vi "Main.vi"() -> ()   [LabVIEW 2019]
uses:
  Motion Profile States.ctl
panel:
  out "CSV (P-V-T)":string[][](table)
  in  "Time between intervals (ms)":dbl=20.0
  in  "Rampdown time (ms)":dbl
  in  "Rampup time (ms)":dbl
  in  "Distance (in)":dbl
  in  "Max Speed (in/sec)":dbl
  out "P-V-A graph":cluster{dbl[], dbl[]}[](graph)
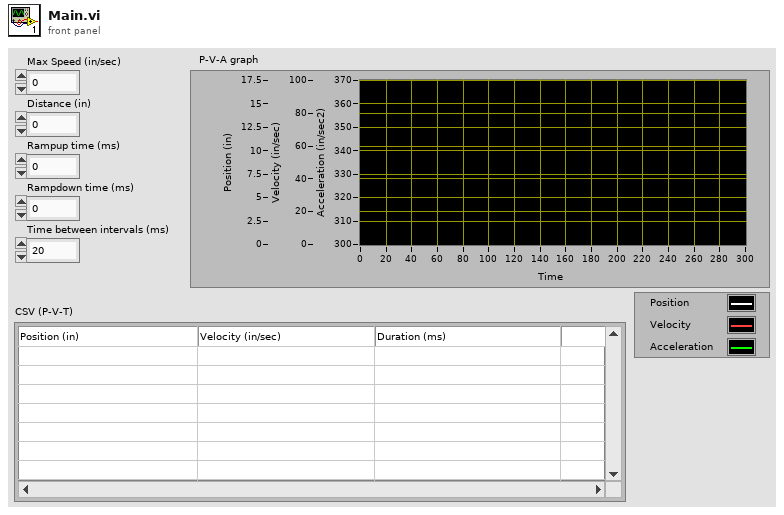
[diagram p1: front panel]
types:
  T1 = typedef "Motion Profile States.ctl" = enum16{"Ramp Up", "ramp down 2", "Steady State", "Ramp Down"}
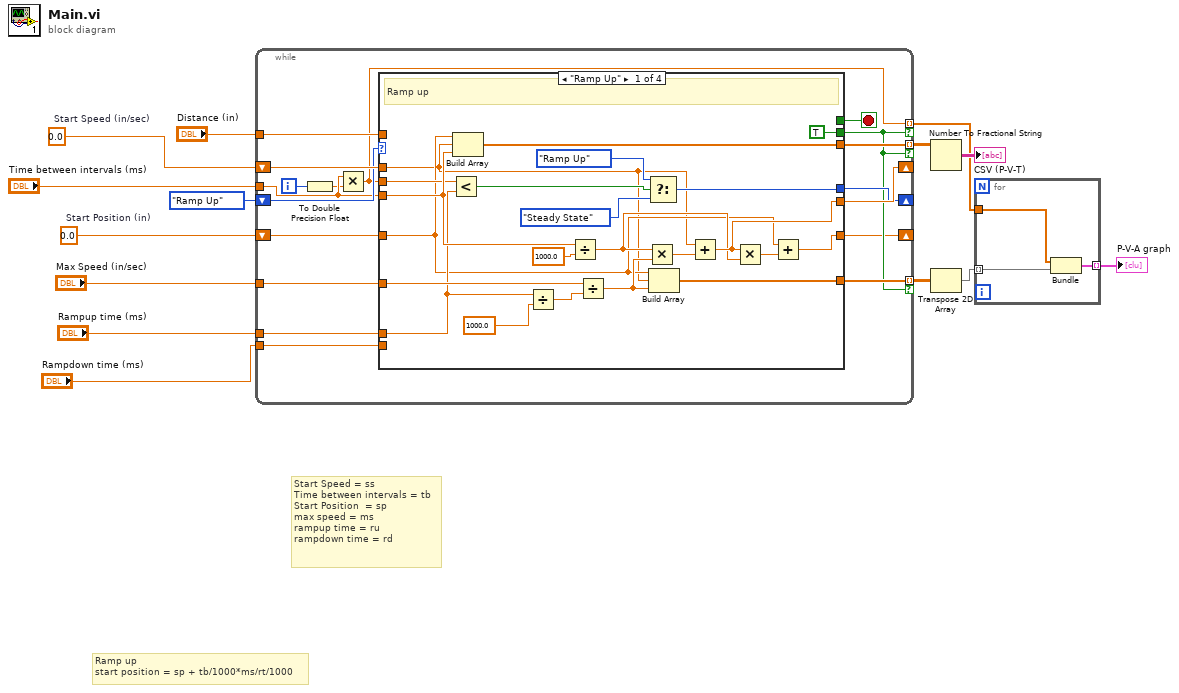
[diagram p0: block diagram]
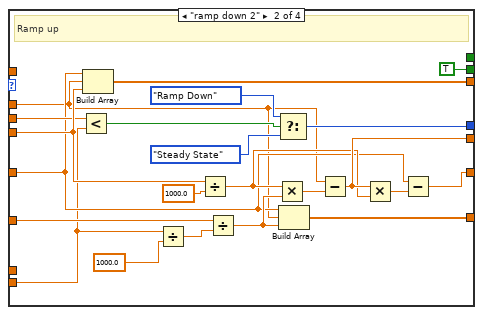
[diagram p2: hidden frame]
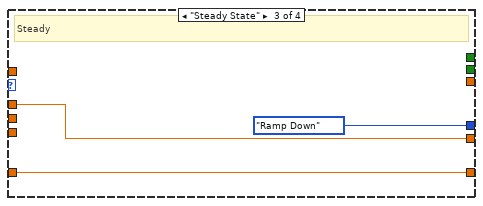
[diagram p3: hidden frame]
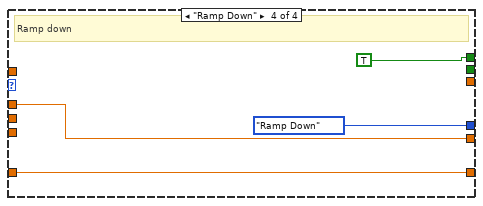
[diagram p4: hidden frame]
diagram:
  w1 = 0.0  # Start Position (in)
  w7 = 0.0  # Start Speed (in/sec)
  # "Ramp up\nstart position = sp + tb/1000*ms/rt/1000"
  # "Start Speed = ss\nTime between intervals = tb\nStart Position  = sp\nmax speed = ms\nrampup time = ru\nrampdown time = rd"
  n1 = while {
    tunnel: "Max Speed (in/sec)" -> [w29]
    tunnel: "Distance (in)" -> [w32]
    tunnel: "Rampup time (ms)" -> [w31]
    tunnel: "Rampdown time (ms)" -> [w30]
    tunnel: "Time between intervals (ms)" -> [w20]
    tunnel: [w28] -> w5 mode=indexing if=w18
    tunnel: [w27] -> w9 mode=indexing if=w18
    shift-right: [w25] -> _
    shift-left: w7 -> [w26]
    shift-right: [w22] -> _
    shift-left: Motion_Profile_States."Ramp Up" -> [w24]
    tunnel: [w17] -> w3 mode=indexing if=w18
    shift-right: [w15] -> _
    shift-left: w1 -> [w16]
    i -> [w21]
    stop <- w23 stop-if-true
    n2 = To Double Precision Float(number=w21) -> (double precision float=w19:dbl)
    n3 = Multiply(x=w20, y=w19) -> (x*y=w17:dbl)
    n4 = case shown="\"Ramp Up\"" w24 {
      tunnel: w32 -> [_ _ _ _]
      tunnel: w31 -> [w42 _ _ _]
      tunnel: w30 -> [_ w55 _ _]
      tunnel: w29 -> [w54 w76 _ _]
      tunnel: w20 -> [w49 w71 _ _]
      tunnel: [w53 w75 _ _] -> w28
      tunnel: [w52 w74 _ _] -> w27
      tunnel: [TRUE TRUE _ _] -> w18
      tunnel: w26 -> [w33 w56 w79 w83]
      tunnel: [w36 w59 w79 w83] -> w25
      tunnel: [_ _ _ TRUE] -> w23
      tunnel: [w46 w68 Motion_Profile_States."Ramp Down" Motion_Profile_States."Ramp Down"] -> w22
      tunnel: w17 -> [w43 w65 _ _]
      tunnel: w16 -> [w34 w57 w77 w80]
      tunnel: [w39 w62 w77 w80] -> w15
      frame "Ramp Up" {
        # "Ramp up"
        n5 = Less?(x=w43, y=w42) -> (x < y?=w44:bool)
        n6 = Build Array(w34, w33, w49) -> (w52:dbl[])
        n7 = Divide(x=w42, y=1000.0) -> (x/y=w41:dbl)
        n8 = Divide(x=w49, y=1000.0) -> (x/y=w35:dbl)
        n9 = Divide(x=w54, y=w41) -> (x/y=w48:dbl)
        n10 = Multiply(x=w35, y=w48) -> (x*y=w38:dbl)
        n11 = Select(t=Motion_Profile_States."Ramp Up", s=w44, f=Motion_Profile_States."Steady State") -> (s? t:f=w46:T1)
        n12 = Build Array(w34, w33, w48) -> (w53:dbl[])
        n13 = Add(x=w33, y=w38) -> (x+y=w36:dbl)
        n14 = Multiply(x=w36, y=w35) -> (x*y=w37:dbl)
        n15 = Add(x=w34, y=w37) -> (x+y=w39:dbl)
      }
      frame "ramp down 2" {
        # "Ramp up"
        n16 = Less?(x=w65, y=w55) -> (x < y?=w66:bool)
        n17 = Build Array(w57, w56, w71) -> (w74:dbl[])
        n18 = Divide(x=w55, y=1000.0) -> (x/y=w64:dbl)
        n19 = Divide(x=w71, y=1000.0) -> (x/y=w58:dbl)
        n20 = Divide(x=w76, y=w64) -> (x/y=w70:dbl)
        n21 = Multiply(x=w58, y=w70) -> (x*y=w61:dbl)
        n22 = Select(t=Motion_Profile_States."Ramp Down", s=w66, f=Motion_Profile_States."Steady State") -> (s? t:f=w68:T1)
        n23 = Build Array(w57, w56, w70) -> (w75:dbl[])
        n24 = Subtract(x=w56, y=w61) -> (x-y=w59:dbl)
        n25 = Multiply(x=w59, y=w58) -> (x*y=w60:dbl)
        n26 = Subtract(x=w57, y=w60) -> (x-y=w62:dbl)
      }
      frame "Steady State" {
        # "Steady"
      }
      frame "Ramp Down" {
        # "Ramp down"
      }
    }
  }
  n27 = Number To Fractional String(number=w9) -> (F-format string=→"CSV (P-V-T)":string[][])  [unwired: 3 in]
  n28 = Transpose 2D Array(2D array=w5) -> (transposed array=w4:dbl[][])
  n29 = for {
    tunnel: w4 -> [w86] mode=indexing
    tunnel: w3 -> [w85]
    tunnel: [w84] -> w2 mode=indexing
    n30 = Bundle(w85, w86) -> (w84:cluster{dbl[], dbl[]})  [unwired: 1 in]
  }
  "P-V-A graph" <- w2
